vi "Initialize Instrument.vi"(8 "error in (no error)":errorcluster, 10 "Reset":bool, 11 "Keithley 2000 in":refnum<class "Keithley 2000.lvclass">) -> (0 "error out":errorcluster, 3 "Keithley 2000 out":refnum<class "Keithley 2000.lvclass">)   [LabVIEW 2020, in "Keithley 2000.lvclass"]
uses:
  Keithley 2000.lvclass
  C:/Sandbox/Git_Sandbox/WiSpry Test Framework source code (LV20)/WiSpry Test Framework/Instruments/Instrument.lvclass
  Instrument.lvclass/Instrument.ctl
  <instrlib>/Keithley 2000/Keithley 2000.lvlib
  Instrument.lvclass
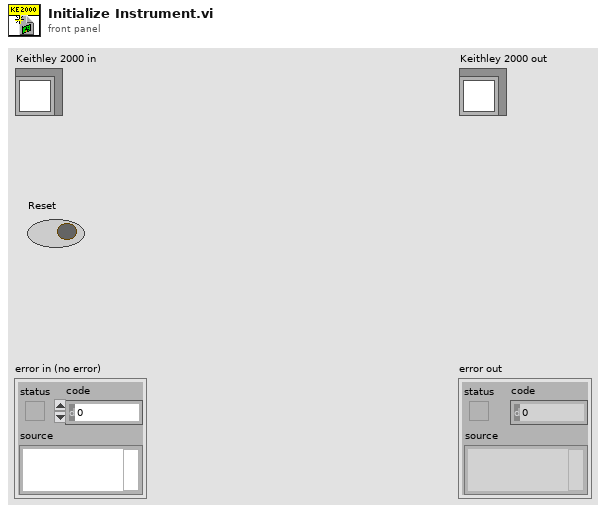
[diagram p1: front panel]
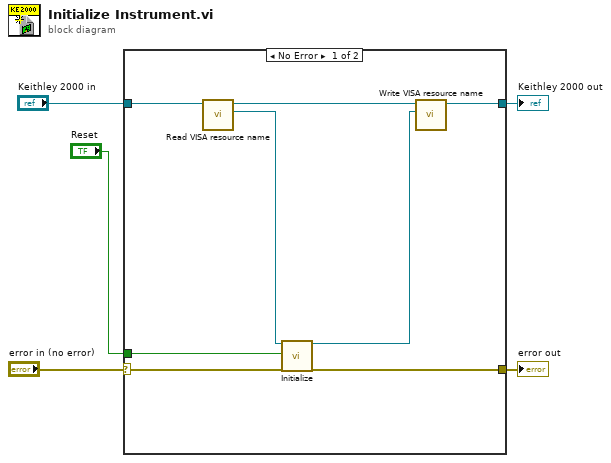
[diagram p0: block diagram]
diagram:
  n1 = case shown="No Error" "error in (no error)" {
    selector: "error in (no error)" -> [w13 w15]
    tunnel: [w12 w15] -> w4
    tunnel: "Keithley 2000 in" -> [w11 w14]
    tunnel: [w9 w14] -> w2
    tunnel: "Reset" -> [w6 _]
    frame No Error {
      n2 = call "Read VISA resource name.vi"("Instrument in"=w11) -> ("VISA resource name"=w7:refnum<visa-resource-name>, "Instrument out"=w10:refnum<class "Keithley 2000.lvclass">)  [unwired: 9 in]
      n3 = call <instrlib>:"Initialize.vi"("VISA resource name"=w7, "Reset? (T: Reset)"=w6, "error in (no error)"=w13) -> ("VISA resource name out"=w8:refnum<visa-resource-name>, "error out"=w12:errorcluster)  [unwired: 15 in]
      n4 = call "Write VISA resource name.vi"("VISA resource name"=w8, "Instrument in"=w10) -> ("Instrument out"=w9:refnum<class "Keithley 2000.lvclass">)  [unwired: 9 in]
    }
    frame Error {
    }
  }
  "error out" <- w4
  "Keithley 2000 out" <- w2
